vi "Parse Project.vi"(8 "Error In":errorcluster, 9 "External Target Map":map{string, string}(c390), 10 "Internal Target Map":map{string, string}(c390), 11 "Project Path in":path) -> (0 "Error Out":errorcluster, 1 "Found External dependencies":string[](array[string]), 2 "Found Internal Dependencies":string[](array[string]), 3 "Project Path dub":path)   [LabVIEW 2019]
doc: "Parse a project file for internal and external dependencies.\n\nInternal dependencies are expected to have 'paths' like vi.lib\\...\nExternal dependencies are identified by unique folder names.\n\n2020-11-11: Henrik Dueholm Hansen"
uses:
  e524974c-34eb-4671-beff-d851fc979908.vi
  be0d84c9-e7ab-4411-bc6b-938b67c5239a.vi
  c89a1cd9-d7f9-4415-bfd9-9928ae79c8ba.vi
  1c34d1f9-9cd2-45b5-a580-df1c6381156c.vi
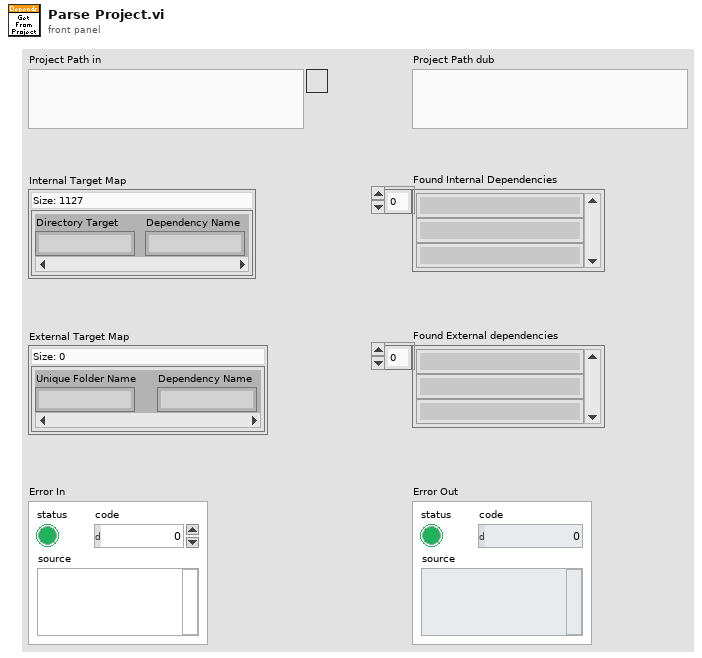
[diagram p1: front panel]
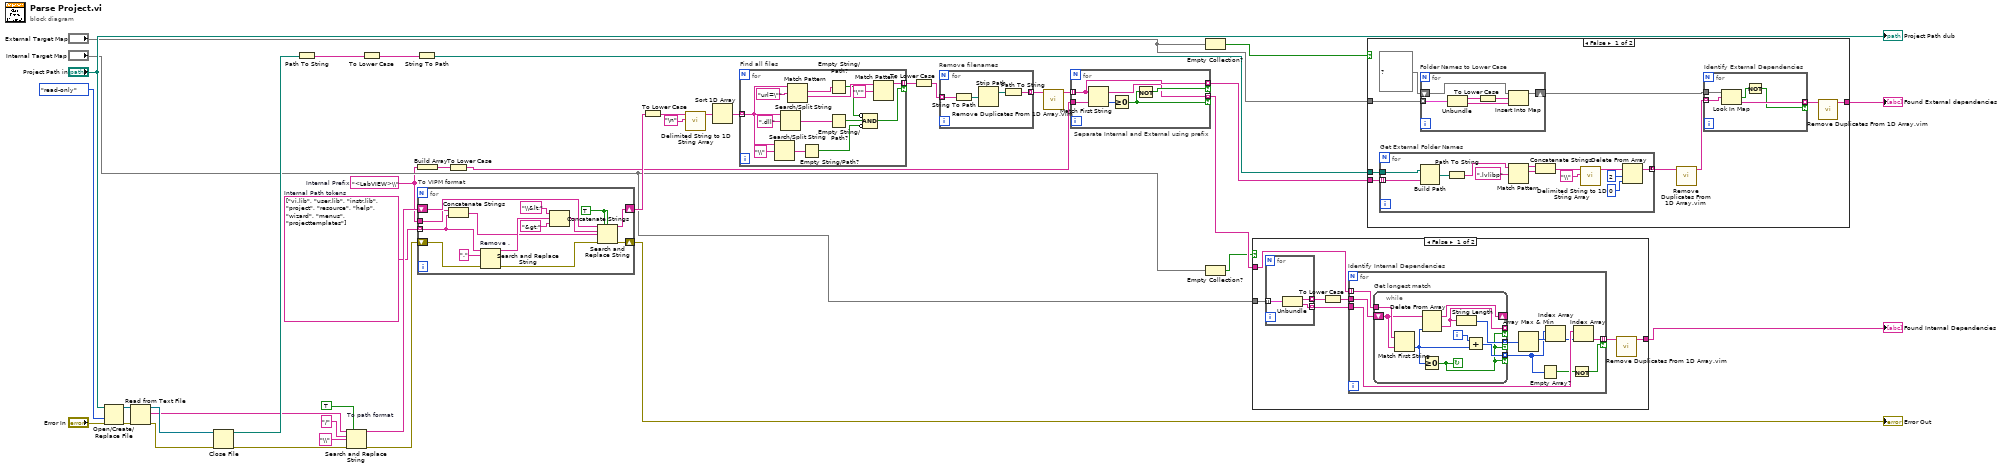
[diagram p0: block diagram]
diagram:
  w1 = "<LabVIEW>\\"  # Internal Prefix
  w15 = string[] ["vi.lib", "user.lib", "instr.lib", "project", "resource", "help", "wizard", "menus", "projecttemplates"]  # Internal Path tokens
  n1 = Open/Create/Replace File(file path (use dialog)="Project Path in", error in="Error In", access (0:read/write)=enum16{"read/write", "read-only", "write-only"}."read-only") -> (refnum out=w39:refnum<file>, error out=w38:errorcluster)  [unwired: 3 in, 1 out]
  n2 = Read from Text File(file (use dialog)=w39, error in=w38) -> (refnum out=w37:refnum<file>, text=w22:string, error out=w36:errorcluster)  [unwired: 2 in, 1 out]
  n3 = Close File(refnum=w37, error in=w36) -> (path=w23:path, error out=w17:errorcluster)
  n4 = Path To String(path=w23) -> (string=w25:string)
  n5 = Search and Replace String "To path format"(replace all?=TRUE ("replace all? (F)"), input string=w22, search string="/" ("String"), replace string="\\" ("replace string (\"\")"), error in=w17) -> (result string=w21:string, error out=w16:errorcluster)  [unwired: 3 in, 2 out]
  n6 = To Lower Case(string=w25) -> (all lower case string=w24:string)
  n7 = String To Path(string=w24) -> (path=w11:path)
  n8 = Build Array(w1) -> (w3:string[])
  n9 = for "To VIPM format" {
    shift-right: [w53] -> w35
    shift-left: w21 -> [w54]
    shift-right: [w52] -> w33
    shift-left: w16 -> [w43]
    tunnel: w15 -> [w45] mode=indexing
    tunnel: w1 -> [w41]
    w51 = TRUE ("replace all? (F)")
    n10 = Concatenate Strings(w41, w45) -> (w44:string)
    n11 = Search and Replace String "Remove ."(input string=w45, search string="." ("String"), error in=w43) -> (result string=w49:string, error out=w42:errorcluster)  [unwired: 5 in, 2 out]
    n12 = Concatenate Strings("\\&lt;", w49, "&gt;" ("string")) -> (w46:string)
    n13 = Search and Replace String(replace all?=w51, case sensitive?=w51, input string=w54, search string=w46, replace string=w44, error in=w42) -> (result string=w53:string, error out=w52:errorcluster)  [unwired: 2 in, 2 out]
  }
  "Error Out" <- w33
  n14 = To Lower Case(string=w3) -> (all lower case string=w2:string[])
  n15 = To Lower Case(string=w35) -> (all lower case string=w30:string)
  n16 = call <vilib>:"Delimited String to 1D String Array.vi"("delimiter"="\n", "delimited string"=w30) -> ("string array"=w28:string[])  [unwired: 9 in]
  n17 = Sort 1D Array(array=w28) -> (sorted array=w34:string[])
  n18 = for "Find all files" {
    tunnel: w34 -> [w61] mode=indexing
    tunnel: [w57] -> w32 mode=indexing if=w56
    n19 = Search/Split String(string=w61, search string/char (-)="\\") -> (match + rest of string=w59:string)  [unwired: 1 in, 2 out]
    n20 = Search/Split String(string=w61, search string/char (-)=".dll") -> (match + rest of string=w65:string)  [unwired: 1 in, 2 out]
    n21 = Match Pattern(string=w61, regular expression="url=\"") -> (match substring=w67:string, after substring=w66:string)  [unwired: 1 in, 2 out]
    n22 = Empty String/Path?(string/path=w59) -> (empty?=w58:bool)
    n23 = Empty String/Path?(string/path=w67) -> (empty?=w62:bool)
    n24 = Empty String/Path?(string/path=w65) -> (empty?=w63:bool)
    n25 = Compound Arithmetic op=AND(invert w62, w63, invert w58) -> (w56:bool)
    n26 = Match Pattern(string=w66, regular expression="\"") -> (before substring=w57:string)  [unwired: 1 in, 3 out]
  }
  n27 = To Lower Case(string=w32) -> (all lower case string=w26:string[])
  n28 = for "Remove filenames" {
    tunnel: w26 -> [w72] mode=indexing
    tunnel: [w69] -> w27 mode=indexing
    n29 = String To Path(string=w72) -> (path=w71:path)
    n30 = Strip Path(path=w71) -> (stripped path=w70:path)  [unwired: 1 out]
    n31 = Path To String(path=w70) -> (string=w69:string)
  }
  n32 = call "Remove Duplicates From 1D Array.vim"("array"=w27) -> ("array with duplicates removed"=w14:string[])  [unwired: 10 in]
  n33 = for "Separate Internal and External using prefix" {
    tunnel: w14 -> [w76] mode=indexing
    tunnel: [w73] -> w13 mode=indexing if=w77
    tunnel: [w76] -> w10 mode=indexing if=w75
    tunnel: w2 -> [w74]
    n34 = Match First String(2:w74, 3:w76) -> (0:w78:i32, 1:w73:string)
    n35 = Greater Or Equal To 0?(x=w78) -> (x >= 0?=w77:bool)
    n36 = Not(x=w77) -> (.not. x?=w75:bool)
  }
  n37 = Empty Collection?(1:"External Target Map") -> (0:w4:bool)
  n38 = Empty Collection?(1:"Internal Target Map") -> (0:w6:bool)
  n39 = case shown="False" w6 {
    tunnel: w13 -> [w84 _]
    tunnel: [w80 _] -> w12
    tunnel: "Internal Target Map" -> [w79 _]
    frame False {
      n40 = for {
        tunnel: w79 -> [w107] mode=indexing
        tunnel: [w106] -> w85 mode=indexing
        tunnel: [w105] -> w82 mode=indexing
        n41 = Unbundle(w107) -> ("Directory Target"=w106:string, "Dependency Name"=w105:string)
      }
      n42 = To Lower Case(string=w85) -> (all lower case string=w83:string[])
      n43 = for "Identify Internal Dependencies" {
        tunnel: w84 -> [w95] mode=indexing
        tunnel: [w92] -> w81 mode=indexing if=w86
        tunnel: w83 -> [w94]
        tunnel: w82 -> [w93]
        n44 = while "Get longest match" {
          tunnel: w95 -> [w104]
          shift-right: [w101] -> _
          shift-left: w94 -> [w103]
          tunnel: [w100] -> w88 mode=indexing if=w96
          tunnel: [w98] -> _ mode=indexing if=w96
          tunnel: [w97] -> w91 mode=indexing if=w96
          i -> [w99]
          stop <- w96 continue-if-true
          n45 = Match First String(2:w103, 3:w104) -> (0:w102:i32)  [unwired: 1 out]
          n46 = Delete From Array(array=w103, index=w102) -> (deleted portion=w98:string, array with subset deleted=w101:string[])  [unwired: 1 in]
          n47 = Greater Or Equal To 0?(x=w102) -> (x >= 0?=w96:bool)
          n48 = String Length(string=w98) -> (length=w97:i32)
          n49 = Add(x=w99, y=w102) -> (x+y=w100:i32)
        }
        n50 = Array Max & Min(array=w91) -> (max index (indices)=w90:i32)  [unwired: 3 out]
        n51 = Empty Array?(array=w88) -> (empty?=w87:bool)
        n52 = Index Array(array=w88, index=w90) -> (element=w89:i32)
        n53 = Not(x=w87) -> (.not. x?=w86:bool)
        n54 = Index Array(array=w93, index=w89) -> (element=w92:string)
      }
      n55 = call "Remove Duplicates From 1D Array.vim"("array"=w81) -> ("array with duplicates removed"=w80:string[])  [unwired: 10 in]
    }
    frame True {
    }
  }
  "Found Internal Dependencies" <- w12
  n56 = case shown="False" w4 {
    tunnel: "External Target Map" -> [w116 _]
    tunnel: w11 -> [w114 _]
    tunnel: w10 -> [w113 _]
    tunnel: [w108 _] -> w9
    frame False {
      n57 = for "Get External Folder Names" {
        tunnel: w114 -> [w133]
        tunnel: w113 -> [w132] mode=indexing
        tunnel: [w127] -> w112 mode=concatenating
        n58 = Build Path(base path=w133, name or relative path=w132) -> (appended path=w134:path)
        n59 = Path To String(path=w134) -> (string=w125:string)
        n60 = Match Pattern(string=w125, regular expression=".lvlibp") -> (before substring=w124:string, match substring=w122:string)  [unwired: 1 in, 2 out]
        n61 = Concatenate Strings(w124, w122) -> (w123:string)
        n62 = call <vilib>:"Delimited String to 1D String Array.vi"("delimiter"="\\" ("search string/char (-)"), "delimited string"=w123) -> ("string array"=w131:string[])  [unwired: 9 in]
        n63 = Delete From Array(array=w131, length=2, index=0) -> (array with subset deleted=w127:string[])  [unwired: 1 out]
      }
      n64 = for "Folder Names to Lower Case" {
        tunnel: w116 -> [w140] mode=indexing
        shift-right: [w137] -> w110
        shift-left: map{string, string} {} ("External Target Map") -> [w138]
        n65 = Unbundle(w140) -> ("Unique Folder Name"=w139:string, "Dependency Name"=w135:string)
        n66 = To Lower Case(string=w139) -> (all lower case string=w136:string)
        n67 = Insert Into Map(map in=w138, key=w136, value=w135) -> (map out=w137:map{string, string})  [unwired: 2 out]
      }
      n68 = call "Remove Duplicates From 1D Array.vim"("array"=w112) -> ("array with duplicates removed"=w111:string[])  [unwired: 10 in]
      n69 = for "Identify External Dependencies" {
        tunnel: w111 -> [w120] mode=indexing
        tunnel: w110 -> [w121]
        tunnel: [w118] -> w109 mode=indexing if=w117
        n70 = Look In Map(map=w121, key=w120) -> (key not found?=w119:bool, value=w118:string)  [unwired: 1 in]
        n71 = Not(x=w119) -> (.not. x?=w117:bool)
      }
      n72 = call "Remove Duplicates From 1D Array.vim"("array"=w109) -> ("array with duplicates removed"=w108:string[])  [unwired: 10 in]
    }
    frame True {
    }
  }
  "Found External dependencies" <- w9
  "Project Path dub" <- "Project Path in"
